vi "New Card Set Up.vi"(8 "Wiring Strings And Values []":T1, 9 "Current Strings And Values []":T1, 10 "Card Array":bool[](array[boolean]), 11 "Voltage Strings And Values []":T1) -> (0 "Current number select":u16, 1 "Time Cluster":T2, 2 "Voltage Number Select":u16, 3 "Continuous?":bool, 4 "Card chosen":i32, 5 "Data Logging Interval 2":u16=1 min=1 step=1 format="%<%H:%M:%S>t", 6 "Wiring (0: 1P2W, 1P2W, 1P2W) 2":u16(ring) items=["1P2W, 1P2W, 1P2W", "1P3W, 1P2W", "3P3W, 1P2W", "1P2W, 1P3W", "1P2W, 3P3W", "3P4W", "3V3A"])   [LabVIEW 2013, in "Universal Power Meter.lvlib" / "Universal Card.lvclass"]
uses:
  Universal Card.lvclass
  Controls/Numeric Time.ctl
  <vilib>/Utility/miscctls.llb/LVStringsAndValuesArrayTypeDef_U16.ctl
panel:
  in  "Wiring":u16(ring) items=["1P3W", "3P3W", "3P4W", "3V3A"]
  in  "Data Logging Interval":u16=1 min=1 step=1 format="%<%H:%M:%S>t"
  in  "Current":u16(ring) items=["Auto", "5mA", "10mA", "20mA", "50mA", "100mA", "200mA", "0.5A", "1A", "2A", "5A", "10A", "20A", "50mV", "100mV", "200mV", "2.5V", "5V", "10V"]
  in  "Voltage":u16(ring) items=["Auto", "15V", "30V", "60V", "150V", "300V", "600V"]
  in  "Play Button":bool
  in  "Card to Start":u16(ring) items=["1"]
  in  "Measurement":enum32{"Continuous", "Timed"}(radio)
  in  "Measurement Time":T3 format="%<%H:%M:%S>t"
  in  "Warm Up Time":dbl format="%<%H:%M:%S>t"
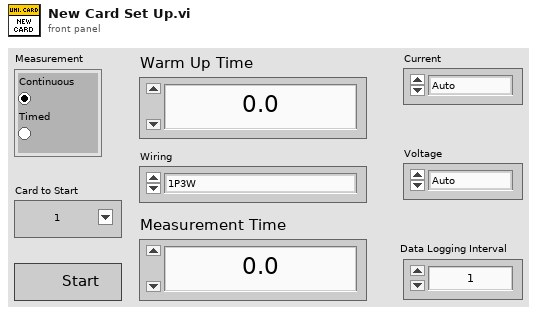
[diagram p1: front panel]
types:
  T1 = typedef "LVStringsAndValuesArrayTypeDef_U16.ctl" = cluster{"String":string, "Value":u16}[]
  T2 = cluster{"Warm Up Time":dbl, "Measurement Time":dbl}
  T3 = typedef "Numeric Time.ctl" = dbl
  T4 = cluster{"Warm Up Time":dbl, "Measurement Time":T3}
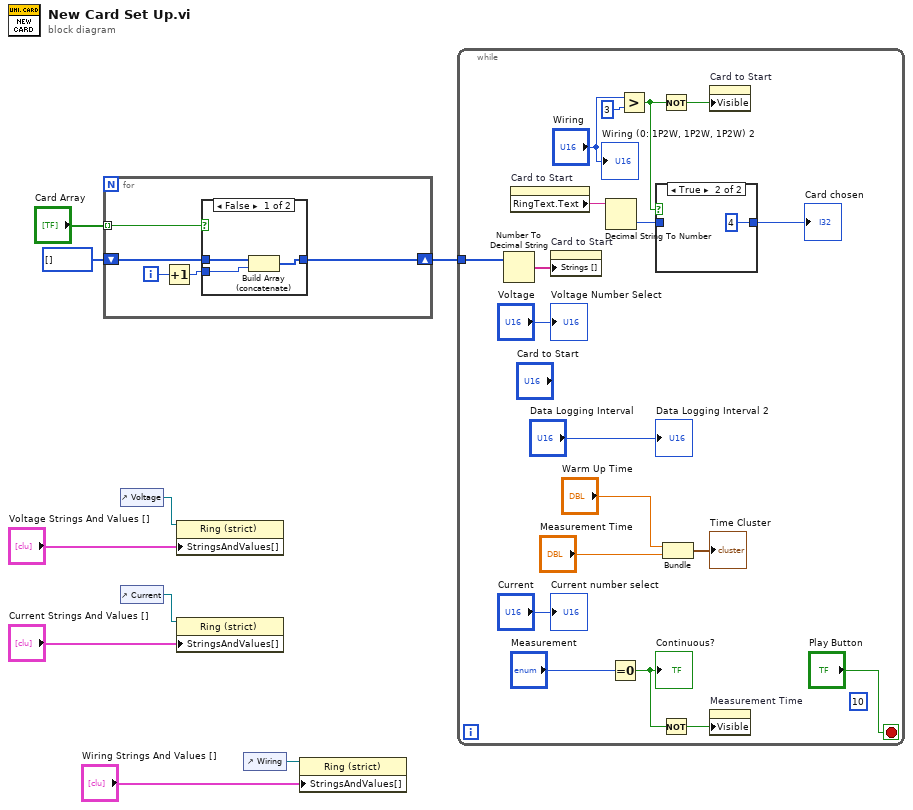
[diagram p0: block diagram]
diagram:
  n1 = for {
    tunnel: "Card Array" -> [w14] mode=indexing
    shift-right: [w10] -> w7
    shift-left: i32[] [] -> [w13]
    i -> [w12]
    n2 = Increment(x=w12) -> (x+1=w11:i32)
    n3 = case shown="False" w14 {
      tunnel: w13 -> [w17 w18]
      tunnel: w11 -> [w16 _]
      tunnel: [w15 w18] -> w10
      frame False {
        n4 = Build Array (concatenate)(w17, w16) -> (w15:i32[])
      }
      frame True {
      }
    }
  }
  n5 = control-ref of="Voltage"() -> (w6:refnum<vi>)
  n6 = control-ref of="Current"() -> (w4:refnum<vi>)
  n7 = property class="Ring (strict)"(reference=w6, "StringsAndValues[]"="Voltage Strings And Values []") -> ()  [unwired: 1 in, 2 out]
  n8 = property class="Ring (strict)"(reference=w4, "StringsAndValues[]"="Current Strings And Values []") -> ()  [unwired: 1 in, 2 out]
  n9 = control-ref of="Wiring"() -> (w2:refnum<vi>)
  n10 = property class="Ring (strict)"(reference=w2, "StringsAndValues[]"="Wiring Strings And Values []") -> ()  [unwired: 1 in, 2 out]
  n11 = while {
    tunnel: w7 -> [w37]
    stop <- "Play Button" stop-if-true
    (unwired) 10
    n12 = Number To Decimal String(number=w37) -> (decimal integer string=w36:string[])  [unwired: 1 in]
    n13 = property on="Card to Start" class="Ring (strict)"() -> ("RingText.Text"=w31:string)  [unwired: 2 in, 2 out]
    n14 = property on="Card to Start" class="Ring (strict)"("Strings []"=w36) -> ()  [unwired: 2 in, 2 out]
    n15 = Decimal String To Number(string=w31) -> (number=w21:i32)  [unwired: 2 in, 1 out]
    n16 = Equal To 0?(x="Measurement") -> (x = 0?=w35:bool)
    "Continuous?" <- w35
    n17 = Greater?(x="Wiring", y=u16 3) -> (0:w22:bool)
    n18 = case shown="True" w22 {
      tunnel: w21 -> [w38 _]
      tunnel: [w38 4] -> w19
      frame False {
      }
      frame True {
      }
    }
    "Card chosen" <- w19
    n19 = Not(x=w22) -> (.not. x?=w24:bool)
    n20 = Not(x=w35) -> (.not. x?=w29:bool)
    n21 = Bundle("Warm Up Time"="Warm Up Time", "Measurement Time"="Measurement Time") -> (→"Time Cluster":T4)  [unwired: 1 in]
    n22 = property on="Card to Start" class="Ring (strict)"("Visible"=w24) -> ()  [unwired: 2 in, 2 out]
    n23 = property on="Measurement Time" class="DigNum (strict)"("Visible"=w29) -> ()  [unwired: 2 in, 2 out]
    "Current number select" <- "Current"
    "Voltage Number Select" <- "Voltage"
    "Data Logging Interval 2" <- "Data Logging Interval"
    "Wiring (0: 1P2W, 1P2W, 1P2W) 2" <- "Wiring"
  }
